vi "ROVOM_VI.vi"() -> ()   [LabVIEW 2018]
panel:
  in  "angle_input":dbl
  out "angle_output _calculated":dbl(knob) scale=-90.0..90.0
  out "angle_output_calculated":dbl
  in  "stop":bool
  out "angle_input":dbl
  out "propeller _vertical_force_calculated":dbl
  out "propeller_horizontal_force_calculated":dbl
  in  "angular velocity":dbl
  in  "velocity_magnitude":dbl
  in  "area":dbl
  in  "medium_density":dbl
  in  "drag_coefficient":dbl
  in  "gravitational_constant":dbl
  in  "mass":dbl
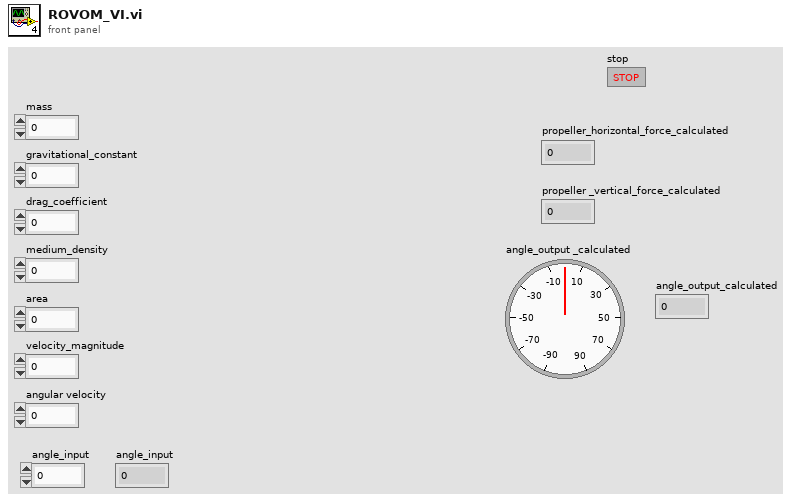
[diagram p1: front panel]
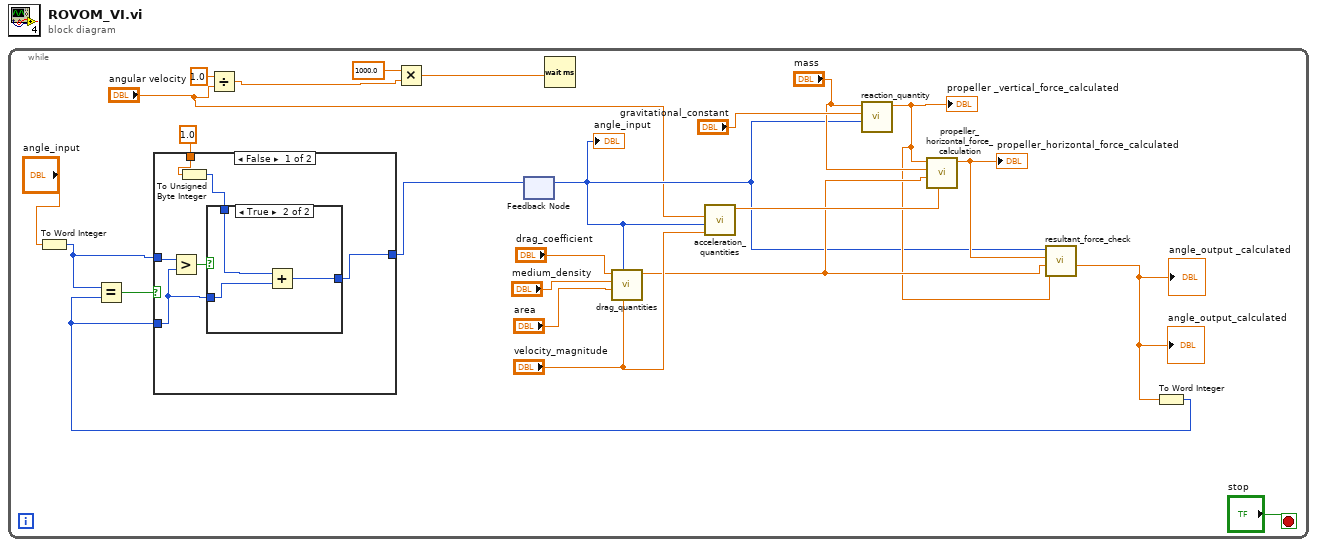
[diagram p0: block diagram]
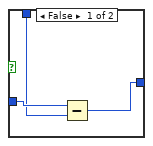
[diagram p2: hidden frame]
diagram:
  n1 = while {
    stop <- "stop" stop-if-true
    n2 = To Word Integer(number="angle_input") -> (16bit integer=w1:i16)
    n3 = Divide(x=1.0, y="angular velocity") -> (x/y=w7:dbl)
    n4 = Multiply(x=1000.0, y=w7) -> (x*y=w10:dbl)
    n5 = feedback #1() -> (w11:i16)  [unwired: 1 in]
    "angle_input" <- w11
    n6 = Wait (ms)(milliseconds to wait=w10) -> ()  [unwired: 1 out]
    n7 = call "drag_quantities.vi"("velocity_magnitude"="velocity_magnitude", "angle_input"=w11, "area"="area", "medium_density"="medium_density", "drag-coefficient"="drag_coefficient") -> ("drag_magnitude"=w15:dbl)  [unwired: 4 in, 2 out]
    n8 = call "acceleration_quantities.vi"("angular_velocity"="angular velocity", "angle_input"=w11, "velocity_magnitude"="velocity_magnitude") -> ("acceleration_magnitude"=w17:dbl)  [unwired: 4 in, 3 out]
    n9 = call "reaction_quantity.vi"("angle_input"=w11, "gravitational_constant"="gravitational_constant", "mass"="mass") -> ("reaction"=w14:dbl)  [unwired: 8 in]
    "propeller _vertical_force_calculated" <- w14
    n10 = call "propeller_horizontal_force_calculation.vi"("acceleration_magnitude"=w17, "drag_magnitude"=w15, "mass"="mass", "reaction"=w14) -> ("propeller_horizontal_force"=w16:dbl)  [unwired: 7 in]
    "propeller_horizontal_force_calculated" <- w16
    n11 = call "resultant_force_check.vi"("reaction"=w14, "drag_magnitude"=w15, "propeller_horizontal_force"=w16, "angle_input"=w11) -> ("angle_out"=w4:dbl)  [unwired: 5 in, 2 out]
    "angle_output_calculated" <- w4
    "angle_output _calculated" <- w4
    n12 = To Word Integer(number=w4) -> (16bit integer=w3:i16)
    n13 = Equal?(x=w1, y=w3) -> (x = y?=w13:bool)
    n14 = case shown="False" w13 {
      tunnel: w1 -> [w30 w37]
      tunnel: [w27 w37] -> w12
      tunnel: w3 -> [w28 _]
      tunnel: 1.0 ("angular velocity") -> [w26 _]
      frame False {
        n15 = Greater?(x=w30, y=w28) -> (0:w29:bool)
        n16 = To Unsigned Byte Integer(number=w26) -> (unsigned 8bit integer=w25:u8)
        n17 = case shown="True" w29 {
          tunnel: w28 -> [w33 w36]
          tunnel: w25 -> [w31 w34]
          tunnel: [w32 w35] -> w27
          frame False {
            n18 = Subtract(x=w33, y=w31) -> (x-y=w32:i16)
          }
          frame True {
            n19 = Add(x=w34, y=w36) -> (x+y=w35:i16)
          }
        }
      }
      frame True {
      }
    }
    n20 = feedback-in #1(w12) -> ()
  }
